vi "4.5.vi"() -> ()   [LabVIEW 2017]
panel:
  out "二维图片":picture
  out "任务五":picture
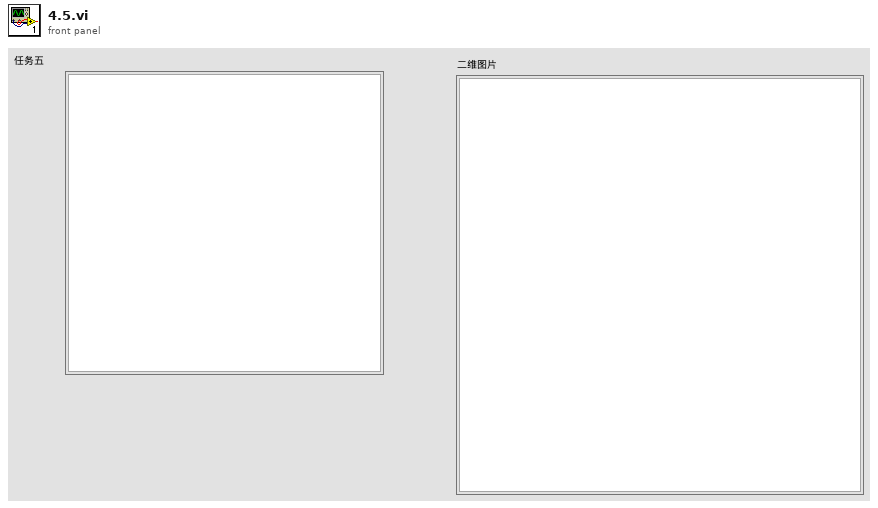
[diagram p1: front panel]
types:
  T1 = typedef "imagedata.ctl" = cluster{"image type":i32, "image depth":i32, "image":u8[], "mask":u8[], "colors":u32[], "Rectangle":cluster{"left":i16, "top":i16, "right":i16, "bottom":i16}}
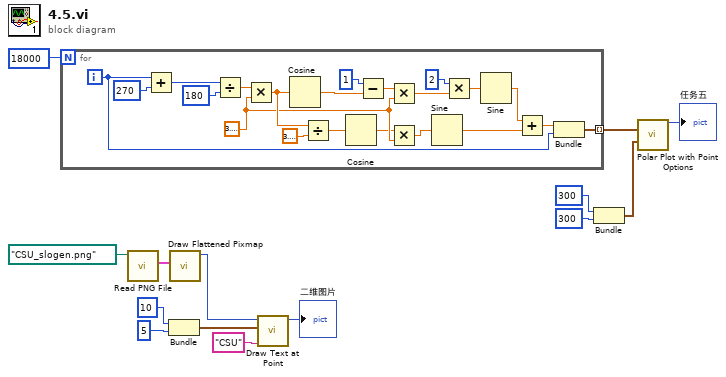
[diagram p0: block diagram]
diagram:
  n1 = for {
    N: 18000 -> [_]
    tunnel: [w33] -> w12 mode=indexing
    i -> [w18]
    w23 = 3.141592653589793
    n2 = Add(x=w18, y=270) -> (x+y=w16:i32)
    n3 = Divide(x=w16, y=180) -> (x/y=w32:dbl)
    n4 = Multiply(x=w32, y=w23) -> (x*y=w27:dbl)
    n5 = Cosine(x=w27) -> (cos(x)=w34:dbl)
    n6 = Divide(x=w27, y=3.141592653589793) -> (x/y=w29:dbl)
    n7 = Cosine(x=w29) -> (cos(x)=w22:dbl)
    n8 = Subtract(x=1, y=w34) -> (x-y=w31:dbl)
    n9 = Multiply(x=w31, y=w23) -> (x*y=w21:dbl)
    n10 = Multiply(x=w22, y=w23) -> (x*y=w30:dbl)
    n11 = Sine(x=w30) -> (sin(x)=w25:dbl)
    n12 = Multiply(x=2, y=w21) -> (x*y=w19:dbl)
    n13 = Sine(x=w19) -> (sin(x)=w26:dbl)
    n14 = Add(x=w26, y=w25) -> (x+y=w24:dbl)
    n15 = Bundle(w24, w18) -> (w33:cluster{dbl, i32})  [unwired: 1 in]
  }
  n16 = call <vilib>:"Read PNG File.vi"("path to PNG file"=path "CSU_slogen.png") -> ("image data"=w7:T1)  [unwired: 8 in, 2 out]
  n17 = Bundle(10, 5) -> (w3:cluster{i32, i32})  [unwired: 1 in]
  n18 = call <vilib>:"Draw Flattened Pixmap.vi"("image data"=w7) -> ("new picture"=w2:picture)  [unwired: 8 in]
  n19 = call <vilib>:"Draw Text at Point.vi"("text"="CSU", "origin"=w3, "picture"=w2) -> ("new picture"=→"二维图片":picture)  [unwired: 7 in, 1 out]
  n20 = Bundle(300, 300) -> (w9:cluster{i32, i32})  [unwired: 1 in]
  n21 = call <vilib>:"Polar Plot with Point Options.vi"("data array [mag, phase (deg)]"=w12, "dimensions (w,h)"=w9) -> ("new picture"=→"任务五":picture)  [unwired: 13 in]
